vi "Tosca-Process AI Color Change.vi"(0 "state in":T1, 1 "Legend":refnum<vi>, 2 "VI in":refnum<vi>, 7 "Row":i32) -> (4 "state out":T1)   [LabVIEW 2020]
uses:
  Typedefs/Tosca-AI UI State.ctl
  Typedefs/Tosca-AI Plot Properties.ctl
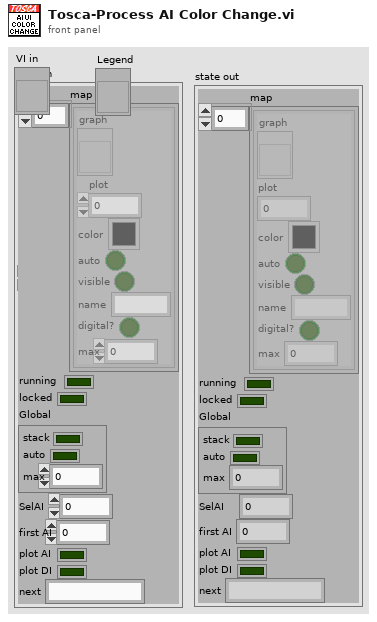
[diagram p1: front panel]
types:
  T1 = typedef "Tosca-AI UI State.ctl" = cluster{"map":T2[], "running":bool, "locked":bool, "Global":cluster{"stack":bool, "auto":bool, "max":dbl}, "SelAI":i32, "first AI":i32, "plot AI":bool, "plot DI":bool, "next":string}
  T2 = typedef "Tosca-AI Plot Properties.ctl" = cluster{"graph":refnum<vi>, "plot":i32, "color":u32, "auto":bool, "visible":bool, "name":string, "digital?":bool, "max":dbl}
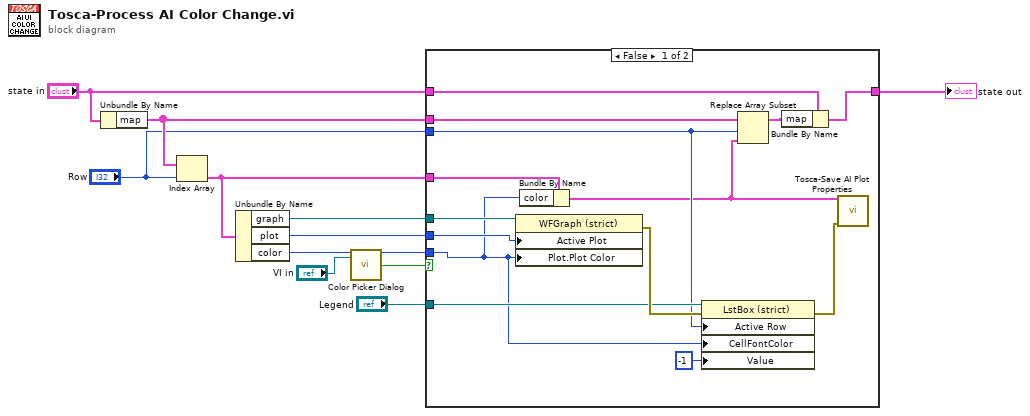
[diagram p0: block diagram]
diagram:
  n1 = Unbundle By Name("state in") -> ("map"=w7:T2[])
  n2 = Index Array(array=w7, index="Row") -> (element=w8:T2)
  n3 = Unbundle By Name(w8) -> ("graph"=w10:refnum<vi>, "plot"=w9:i32, "color"=w12:u32)
  n4 = call "Color Picker Dialog.vi"("Color In"=w12, "parent"="VI in") -> ("Color Out"=w2:u32, "Canceled?"=w1:bool)  [unwired: 12 in]
  n5 = case shown="False" w1 {
    tunnel: w10 -> [w26 _]
    tunnel: w9 -> [w25 _]
    tunnel: w8 -> [w24 _]
    tunnel: w7 -> [w23 _]
    tunnel: "state in" -> [w22 w27]
    tunnel: [w20 w27] -> w5
    tunnel: "Legend" -> [w18 _]
    tunnel: "Row" -> [w17 _]
    tunnel: w2 -> [w16 _]
    frame False {
      n6 = property class="WFGraph (strict)"(reference=w26, "Active Plot"=w25, "Plot.Plot Color"=w16) -> (error out=w19:errorcluster)  [unwired: 1 in, 1 out]
      n7 = Bundle By Name(cluster=w24, "color"=w16) -> (w14:T2)
      n8 = property class="LstBox (strict)"(reference=w18, error in=w19, "Active Row"=w17, "CellFontColor"=w16, "Value"=-1) -> (error out=w13:errorcluster)  [unwired: 1 out]
      n9 = Replace Array Subset(array=w23, new element=w14, index=w17) -> (w21:T2[])
      n10 = Bundle By Name(cluster=w22, "map"=w21) -> (w20:T1)
      n11 = call "Tosca-Save AI Plot Properties.vi"("plot"=w14, "error in (no error)"=w13) -> ()  [unwired: 14 in]
    }
    frame True {
    }
  }
  "state out" <- w5
